vi "PH_BeamlineInformation.PC _Powermeter.vi"(0 "i ref in":refnum<vi>, 2 "serviceName":string, 3 "data":i8[](array[numeric]), 4 "not linked?":bool, 5 "error in (no error)":errorcluster) -> (14 "i ref out":refnum<vi>, 19 "error out":errorcluster)   [LabVIEW 2014, in "PH_BeamlineInformation.lvlib"]
doc: "This VI writes the powermeter values to own attributess"
uses:
  PH_BeamlineInformation.lvlib
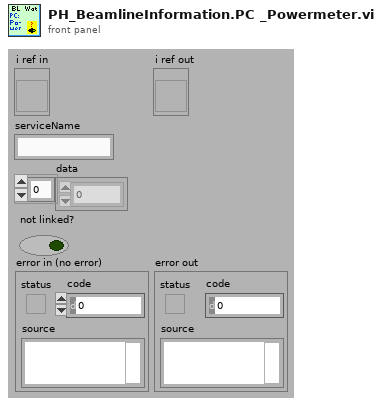
[diagram p1: front panel]
types:
  T1 = typedef "PH_BeamlineInformation.lvlib/PH_BeamlineInformation.i attribute.ctl" = cluster{"BL GUI Elements of Services":cluster{"Service Name":string, "GUI Elements":refnum<vi>[], "Status":i32}[], "Powermeters":T2, "Efficiency":T3, "Heads":T4[]}
  T2 = typedef "PH_BeamlineInformation.lvlib/PH_BeamlineInformation.Powermeter.ctl" = cluster{"ns FE":cluster{"GUI Ref":refnum<vi>, "Value":dbl}, "fs FE":cluster{"GUI Ref":refnum<vi>, "Value":dbl}, "PA":cluster{"GUI Ref":refnum<vi>, "Value":dbl}, "MA":cluster{"GUI Ref":refnum<vi>, "Value":dbl}, "Z6 green":cluster{"GUI Ref":refnum<vi>, "Value":dbl}, "Z6 IR":cluster{"GUI Ref":refnum<vi>, "Value":dbl}, "Z6 COS":cluster{"GUI Ref":refnum<vi>, "Value":dbl}}
  T3 = typedef "PH_BeamlineInformation.lvlib/PH_BeamlineInformation.Efficiency.ctl" = cluster{"PA Gain":cluster{"GUI Ref":refnum<vi>, "Value":dbl}, "MA Gain":cluster{"GUI Ref":refnum<vi>, "Value":dbl}, "Z6 green Conversion":cluster{"GUI Ref":refnum<vi>, "Value":dbl}, "Z6 Comp Losses":cluster{"GUI Ref":refnum<vi>, "Value":dbl}}
  T4 = typedef "PH_BeamlineInformation.lvlib/PH_BeamlineInformation.Head.ctl" = cluster{"PowerUnit":T5, "in use":cluster{"Value":bool, "GUI Ref":refnum<vi>, "linked":bool}, "voltage":cluster{"Value":dbl, "GUI Ref":refnum<vi>, "linked":bool}}
  T5 = typedef "PH_PP_Common.lvlib/PH_PP_Common.PUs.ctl" = enum16{"no Info", "PA-19mm-1", "PA-19mm-2", "PA-45mm-PILC", "PA-45mm-MAIN", "MA-PU-1", "MA-PU-2", "MA-PU-3", "MA-PU-4", "MA-PU-5", "MA-PU-6", "MA-FR", "MA-PILC", "PA-45mm-DP"}
  T6 = cluster{"[0]":cluster{"GUI Ref":refnum<vi>, "Value":dbl}, "[1]":cluster{"GUI Ref":refnum<vi>, "Value":dbl}, "[2]":cluster{"GUI Ref":refnum<vi>, "Value":dbl}, "[3]":cluster{"GUI Ref":refnum<vi>, "Value":dbl}, "[4]":cluster{"GUI Ref":refnum<vi>, "Value":dbl}, "[5]":cluster{"GUI Ref":refnum<vi>, "Value":dbl}, "[6]":cluster{"GUI Ref":refnum<vi>, "Value":dbl}}
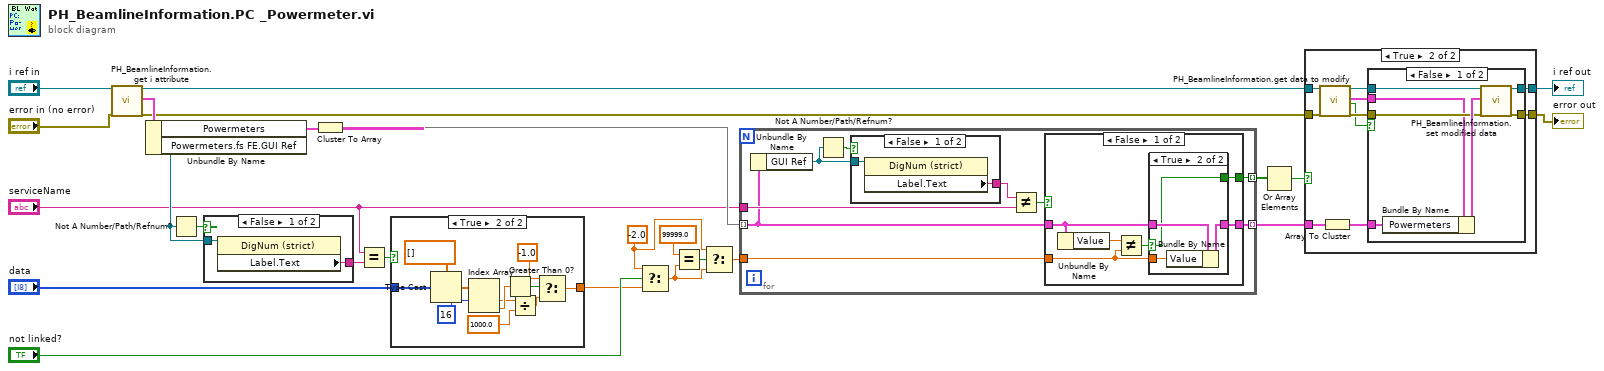
[diagram p0: block diagram]
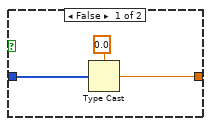
[diagram p2: hidden frame]
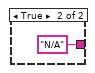
[diagram p3: hidden frame]
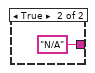
[diagram p6: hidden frame]
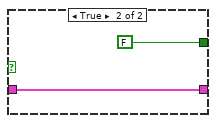
[diagram p8: hidden frame]
diagram:
  w4 = -2.0 ("t")
  n1 = call "PH_BeamlineInformation.get i attribute.vi"("i ref in"="i ref in", "error in (no error)"="error in (no error)") -> ("i ref out"=w21:refnum<vi>, "i attribute"=w25:T1, "error out"=w17:errorcluster)  [unwired: 15 in]
  n2 = Unbundle By Name(w25) -> ("Powermeters"=w22:T2, "Powermeters.fs FE.GUI Ref"=w9:refnum<vi>)
  n3 = Not A Number/Path/Refnum?(number/path/refnum=w9) -> (NaN/Path/Refnum?=w10:bool)
  n4 = case shown="False" w10 {
    tunnel: w9 -> [w27 _]
    tunnel: [w26 "N/A" ("Label.Text")] -> w3
    frame False {
      n5 = property class="DigNum (strict)"(reference=w27) -> ("Label.Text"=w26:string)  [unwired: 1 in, 2 out]
    }
    frame True {
    }
  }
  n6 = Cluster To Array(cluster=w22) -> (array=w14:cluster{"GUI Ref":refnum<vi>, "Value":dbl}[])
  n7 = Equal?(x="serviceName", y=w3) -> (x = y?=w8:bool)
  n8 = case shown="True" w8 {
    tunnel: [w31 w35] -> w5
    tunnel: "data" -> [w30 w42]
    frame False {
      n9 = Type Cast(type=0.0, x=w30) -> (*(type *) &x=w31:dbl)
    }
    frame True {
      n10 = Type Cast(type=dbl[] [], x=w42) -> (*(type *) &x=w40:dbl[])
      n11 = Index Array(array=w40, index #1=16 ("index")) -> (element #1=w34:dbl, element #2=w38:dbl)  [unwired: 1 in]
      n12 = Greater Than 0?(x=w38) -> (x > 0?=w37:bool)
      n13 = Divide(x=w34, y=1000.0) -> (x/y=w32:dbl)
      n14 = Select(t=-1.0, s=w37, f=w32) -> (s? t:f=w35:dbl)
    }
  }
  n15 = Select(t=w4, s="not linked?", f=w5) -> (s? t:f=w6:dbl)
  n16 = Equal?(x=99999.0 ("y"), y=w6) -> (x = y?=w16:bool)
  n17 = Select(t=w4, s=w16, f=w6) -> (s? t:f=w1:dbl)
  n18 = for {
    tunnel: w14 -> [w45] mode=indexing
    tunnel: "serviceName" -> [w50]
    tunnel: [w48] -> w13 mode=indexing
    tunnel: [w44] -> w11 mode=indexing
    tunnel: w1 -> [w43]
    n19 = Unbundle By Name(w45) -> ("GUI Ref"=w46:refnum<vi>)
    n20 = Not A Number/Path/Refnum?(number/path/refnum=w46) -> (NaN/Path/Refnum?=w47:bool)
    n21 = case shown="False" w47 {
      tunnel: w46 -> [w53 _]
      tunnel: [w52 "N/A" ("Label.Text")] -> w51
      frame False {
        n22 = property class="DigNum (strict)"(reference=w53) -> ("Label.Text"=w52:string)  [unwired: 1 in, 2 out]
      }
      frame True {
      }
    }
    n23 = Not Equal?(x=w51, y=w50) -> (x != y?=w49:bool)
    n24 = case shown="False" w49 {
      tunnel: [w55 FALSE] -> w48
      tunnel: w45 -> [w59 w67]
      tunnel: [w60 w67] -> w44
      tunnel: w43 -> [w57 _]
      frame False {
        n25 = Unbundle By Name(w59) -> ("Value"=w58:dbl)
        n26 = Not Equal?(x=w58, y=w57) -> (x != y?=w56:bool)
        n27 = case shown="True" w56 {
          selector: w56 -> [w61 w63]
          tunnel: [w62 w66] -> w60
          tunnel: w59 -> [w62 w65]
          tunnel: w57 -> [_ w64]
          tunnel: [w61 w63] -> w55
          frame False {
          }
          frame True {
            n28 = Bundle By Name(cluster=w65, "Value"=w64) -> (w66:cluster{"GUI Ref":refnum<vi>, "Value":dbl})
          }
        }
      }
      frame True {
      }
    }
  }
  n29 = Or Array Elements(Boolean array=w13) -> (logical OR=w12:bool)
  n30 = case shown="True" w12 {
    tunnel: [w70 w74] -> w20
    tunnel: [w69 w73] -> w19
    tunnel: w21 -> [w70 w76]
    tunnel: w17 -> [w69 w75]
    tunnel: w11 -> [_ w72]
    frame False {
    }
    frame True {
      n31 = call "PH_BeamlineInformation.get data to modify.vi"("i ref in"=w76, "error in (no error)"=w75) -> ("i ref out"=w80:refnum<vi>, "i attribute"=w77:T1, "timed out"=w78:bool, "error out"=w79:errorcluster)  [unwired: 14 in]
      n32 = Array To Cluster(array=w72) -> (cluster=w71:T6)
      n33 = case shown="False" w78 {
        tunnel: [w87 w89] -> w74
        tunnel: w80 -> [w86 w89]
        tunnel: w79 -> [w83 w88]
        tunnel: [w85 w88] -> w73
        tunnel: w77 -> [w82 _]
        tunnel: w71 -> [w81 _]
        frame False {
          n34 = Bundle By Name(cluster=w82, "Powermeters"=w81) -> (w84:T1)
          n35 = call "PH_BeamlineInformation.set modified data.vi"("i ref in"=w86, "i attribute"=w84, "error in (no error)"=w83) -> ("i ref out"=w87:refnum<vi>, "error out"=w85:errorcluster)  [unwired: 15 in]
        }
        frame True {
        }
      }
    }
  }
  "error out" <- w19
  "i ref out" <- w20
